vi "EditComment.vi"(0 "Enable":bool=TRUE, 3 "Comment":string, 5 "error in (no error)":errorcluster) -> (17 "Comment":string, 18 "OK":bool, 19 "error out":errorcluster)   [LabVIEW 2016]
doc: "Displays a standard dialog box that prompts users to enter information, such as a user name and password.\n--------------------\n\nThis Express VI is configured as follows:\n\nMessage to Display to the User:\nThe inputs are: \nText Entry Box: Comment"
panel:
  out "String":string
  in  "Cancel":bool
  in  "OK2":bool
  in  "OK1":bool
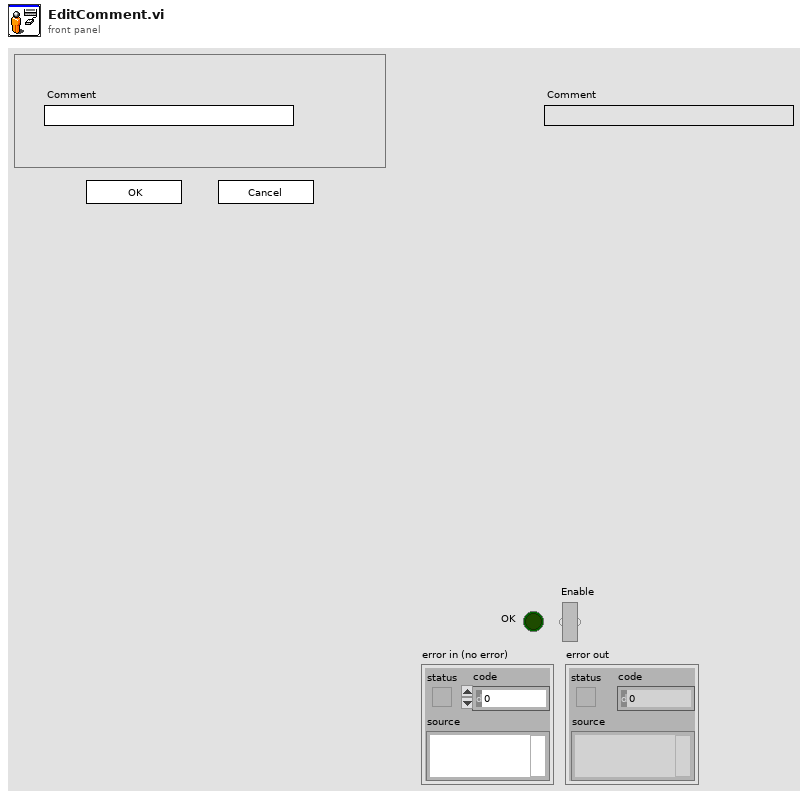
[diagram p1: front panel]
types:
  T1 = cluster{"Input Name":string, "Input Data Type":i32}[]
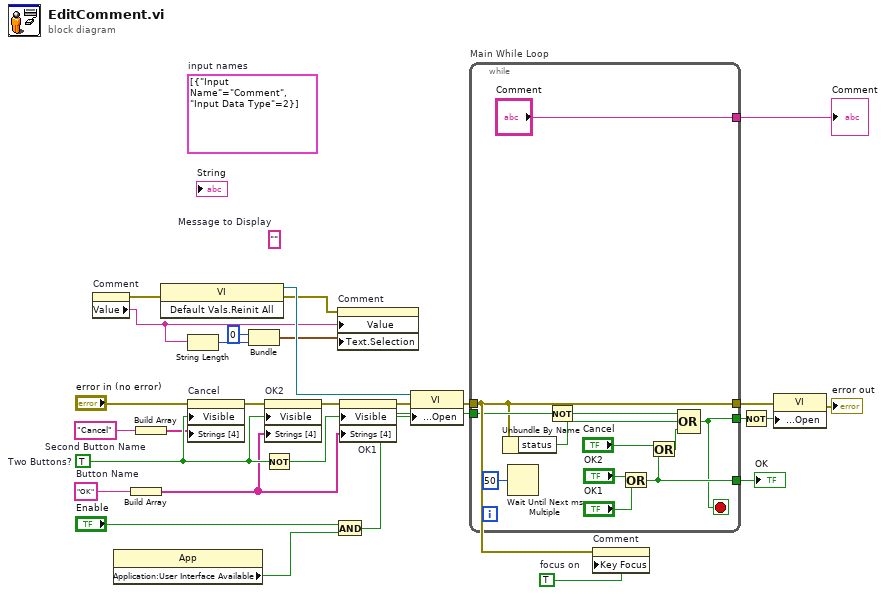
[diagram p0: block diagram]
diagram:
  w7 = TRUE  # focus on
  (unwired) T1 [{"Input Name"="Comment", "Input Data Type"=2}]  # input names
  w20 = "Cancel"  # Second Button Name
  w18 = "OK"  # Button Name
  (unwired) ""  # Message to Display
  w28 = TRUE  # Two Buttons?
  n1 = property on="Comment" class="Str"() -> (error out=w6:errorcluster, "Value"=w4:string)  [unwired: 2 in, 1 out]
  n2 = property class="App"() -> ("Application:User Interface Available"=w10:bool)  [unwired: 2 in, 2 out]
  n3 = Build Array(w18) -> (w19:string[])
  n4 = Build Array(w20) -> (w21:string[])
  n5 = invoke class="VI" method="Default Vals.Reinit All"(error in=w6) -> (reference out=w9:refnum<vi>, error out=w5:errorcluster)  [unwired: 2 in, 1 out]
  n6 = String Length(string=w4) -> (length=w3:i32)
  n7 = property on="Cancel" class="Bool"(error in="error in (no error)", "Visible"=w28, "Strings [4]"=w21) -> (error out=w25:errorcluster)  [unwired: 1 in, 1 out]
  n8 = Bundle(0, w3) -> (w1:cluster{i32, i32})  [unwired: 1 in]
  n9 = Not(x=w28) -> (.not. x?=w26:bool)
  n10 = property on="OK2" class="Bool"(error in=w25, "Visible"=w28, "Strings [4]"=w19) -> (error out=w24:errorcluster)  [unwired: 1 in, 1 out]
  n11 = And(x="Enable", y=w10) -> (x .and. y?=w11:bool)
  n12 = property on="Comment" class="Str"(error in=w5, "Value"=w4, "Text.Selection"=w1) -> ()  [unwired: 1 in, 2 out]
  n13 = property on="OK1" class="Bool"(error in=w24, "Visible"=w26, "Strings [4]"=w19) -> (error out=w17:errorcluster)  [unwired: 1 in, 1 out]
  n14 = property class="VI"(reference=w9, error in=w17, "Front Panel Window:Open"=w11) -> (error out=w16:errorcluster)  [unwired: 1 out]
  n15 = while "Main While Loop" {
    tunnel: [w37] -> w27
    tunnel: w11 -> [w35]
    tunnel: [w33] -> w22
    tunnel: w16 -> [w32]
    tunnel: [w32] -> w14
    tunnel: ["Comment"] -> w8
    stop <- w33 stop-if-true
    n16 = Unbundle By Name(w32) -> ("status"=w30:bool)
    n17 = Wait Until Next ms Multiple(millisecond multiple=u32 50) -> ()  [unwired: 1 out]
    n18 = Not(x=w35) -> (.not. x?=w34:bool)
    n19 = Or(x="OK2", y="OK1") -> (x .or. y?=w37:bool)
    n20 = Or(x="Cancel", y=w37) -> (x .or. y?=w31:bool)
    n21 = Compound Arithmetic op=OR(w34, w30, w31) -> (w33:bool)
  }
  "OK" <- w27
  "Comment" <- w8
  n22 = property on="Comment" class="Str"(error in=w16, "Key Focus"=w7) -> ()  [unwired: 1 in, 2 out]
  n23 = Not(x=w22) -> (.not. x?=w23:bool)
  n24 = property class="VI"(error in=w14, "Front Panel Window:Open"=w23) -> (error out=→"error out":errorcluster)  [unwired: 1 in, 1 out]
